vi "Get_current_comments.vi"() -> (0 "Comment":string)   [LabVIEW 2010]
uses:
  ADAM_Global.vi
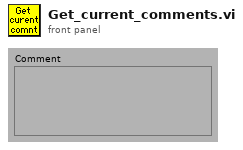
[diagram p1: front panel]
types:
  T1 = typedef "Comments_cluster.ctl" = cluster{"Time":dbl, "Comment":string}
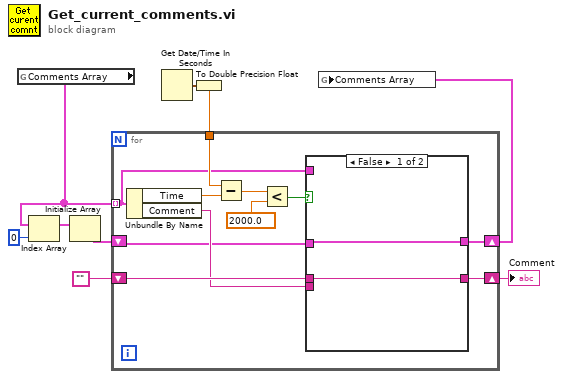
[diagram p0: block diagram]
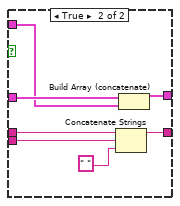
[diagram p2: hidden frame]
diagram:
  n1 = global read "ADAM_Global.vi" "Comments Array"() -> (w3:T1[])
  n2 = Index Array(array=w3, index=0 ("Index")) -> (element=w6:T1)
  n3 = Initialize Array(w6) -> (w5:T1[])  [unwired: 1 out]
  n4 = Get Date/Time In Seconds() -> (seconds since 1Jan1904=w1:timestamp)
  n5 = To Double Precision Float(number=w1) -> (double precision float=w9:dbl)
  n6 = for {
    tunnel: w3 -> [w11] mode=indexing
    shift-right: [w14] -> w2
    shift-left: "" -> [w16]
    tunnel: w9 -> [w20]
    shift-right: [w10] -> w4
    shift-left: w5 -> [w13]
    n7 = Unbundle By Name(w11) -> ("Time"=w12:dbl, "Comment"=w15:string)
    n8 = Subtract(x=w20, y=w12) -> (x-y=w19:dbl)
    n9 = Less?(x=w19, y=2000.0) -> (x < y?=w17:bool)
    n10 = case shown="False" w17 {
      tunnel: w16 -> [w22 w29]
      tunnel: w15 -> [_ w28]
      tunnel: [w22 w26] -> w14
      tunnel: w13 -> [w21 w25]
      tunnel: w11 -> [_ w24]
      tunnel: [w21 w23] -> w10
      frame False {
      }
      frame True {
        n11 = Concatenate Strings(w29, w28, " ") -> (w26:string)
        n12 = Build Array (concatenate)(w25, w24) -> (w23:T1[])
      }
    }
  }
  "Comment" <- w2
  n13 = global write "ADAM_Global.vi" "Comments Array"(w4) -> ()
